vi "AwakeRunner.vi"() -> ()   [LabVIEW 2012]
uses:
  <vilib>/vision/Image Controls.llb/IMAQ Image.ctl
  <vilib>/Platform/TimedLoop/XDataNode/timing_clust.ctl
  <vilib>/Platform/TimedLoop/XDataNode/nitl_modes.ctl
  <vilib>/Platform/TimedLoop/XDataNode/wakeup.ctl
  <instrlib>/niHWS/nihws.llb/niHWS Open File Permissions ID.ctl
  <vilib>/Instr/_visa.llb/Select Event Type.ctl
  <vilib>/DAQmx/write.llb/DAQmx Write (Digital Bool 1Line 1Point).vi
  <vilib>/DAQmx/read.llb/DAQmx Read (Analog Wfm 1Chan NSamp).vi
  <instrlib>/niHWS/nihws.llb/niHWS Write Analog DBL.vi
  <instrlib>/niHWS/nihws.llb/niHWS Write Analog WDT.vi
  <vilib>/DAQmx/miscellaneous.llb/DAQmx Fill In Error Info.vi
  <vilib>/platform/TimedLoop/XDataNode/XDataNode.xnode
  <vilib>/express/express arith-compare/Formula/XNode/ExpressFormulaBlockNode.xnode
  <resource>/objmgr/daqmx.rc
  <vilib>/vision/NI_Vision_Development_Module.lvlib
  <vilib>/ptbypt/NI_PtbyPt.lvlib
  <vilib>/Platform/TimedLoop/XDataNode/XDNodeRunTimeDep.lvlib
panel:
  out "Numeric 2":i32
  out "Numeric":i32
  in  "SyncWrite":bool
  out "Click Value":i8
  out "Image Dst Out":T1
  out "Ephys Rate":dbl=1000.0
  out "Waveform Chart":waveform(dbl)(graph)
  out "Speed History":dbl(graph)
  in  "Magnify":bool
  in  "stop":bool
  out "Camera":T1(plugin-control)
  out "Rec Time":dbl format="%#_3g"
  out "fps":dbl format="%#_2g"
  in  "Rec":bool
  in  "Path":path
  in  "Gain":dbl(slide)=2.6607250597988097 min=1.0 max=3.9810717055349722 scale=0.0..4.0
  in  "Exposure Time":dbl(slide)=16602.0 min=56.0 max=16602.0 scale=0.0..16600.0
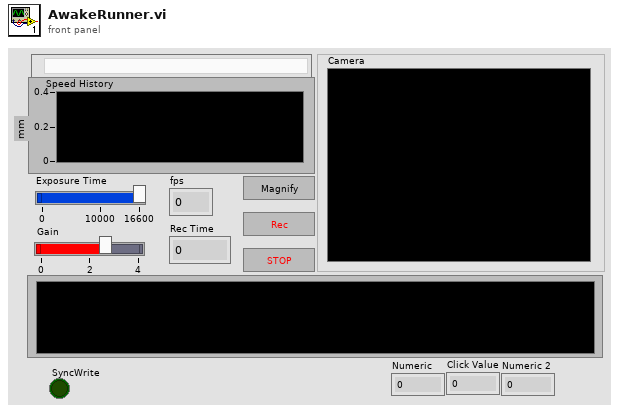
[diagram p1: front panel]
types:
  T1 = typedef "IMAQ Image.ctl" = refnum<image>
  T2 = typedef "XDNodeRunTimeDep.lvlib/timing_clust.ctl" = cluster{"Expected End [f-1]":u64, "Actual End [f-1]":u64, "Finished Late? [f-1]":bool, "Expected End [i-1]":u64, "Actual End [i-1]":u64, "Finished Late? [i-1]":bool, "Expected Start [i]":u64, "Actual Start [i]":u64, "Expected Start [f]":u64, "Actual Start [f]":u64, "Source Name":string, "Structure Name":string, "Period":i64, "Deadline":i64, "Offset":i64, "Start":i64, "Priority":i32, "Timeout":i32, "Mode":T3, "Wakeup Reason":T4, "Error":errorcluster, "Source Type":string, "Secondary Source Type":string, "Global End Time":u64, "Global Start Time":u64, "Frame Duration":u64, "Iteration Duration":u64, "Assigned CPU":i32, "I/O Scan Engine Mode":u32}
  T3 = typedef "XDNodeRunTimeDep.lvlib/nitl_modes.ctl" = enum32{"No Change", "Process missed periods, maintain original phase", "Discard missed periods, maintain original phase", "Process missed periods, ignore original phase", "Discard missed periods, ignore original phase"}
  T4 = typedef "XDNodeRunTimeDep.lvlib/wakeup.ctl" = enum32{"Normal", "Aborted", "Asynchronous wakeup", "Timing source error", "Timed loop error", "Timeout"}
  T5 = enum32{"Invalid", "Standard", "Closed", "Hidden", "Minimized", "Maximized"}
  T6 = typedef "niHWS Open File Permissions ID.ctl" = enum32{"Read Only", "Read/Write Existing", "Read/Write/Create New", "Read/Write/Create New Always"}
  T7 = typedef "AviRefnum.ctl" = refnum<k1>
  T8 = typedef "Select Event Type.ctl" = u32
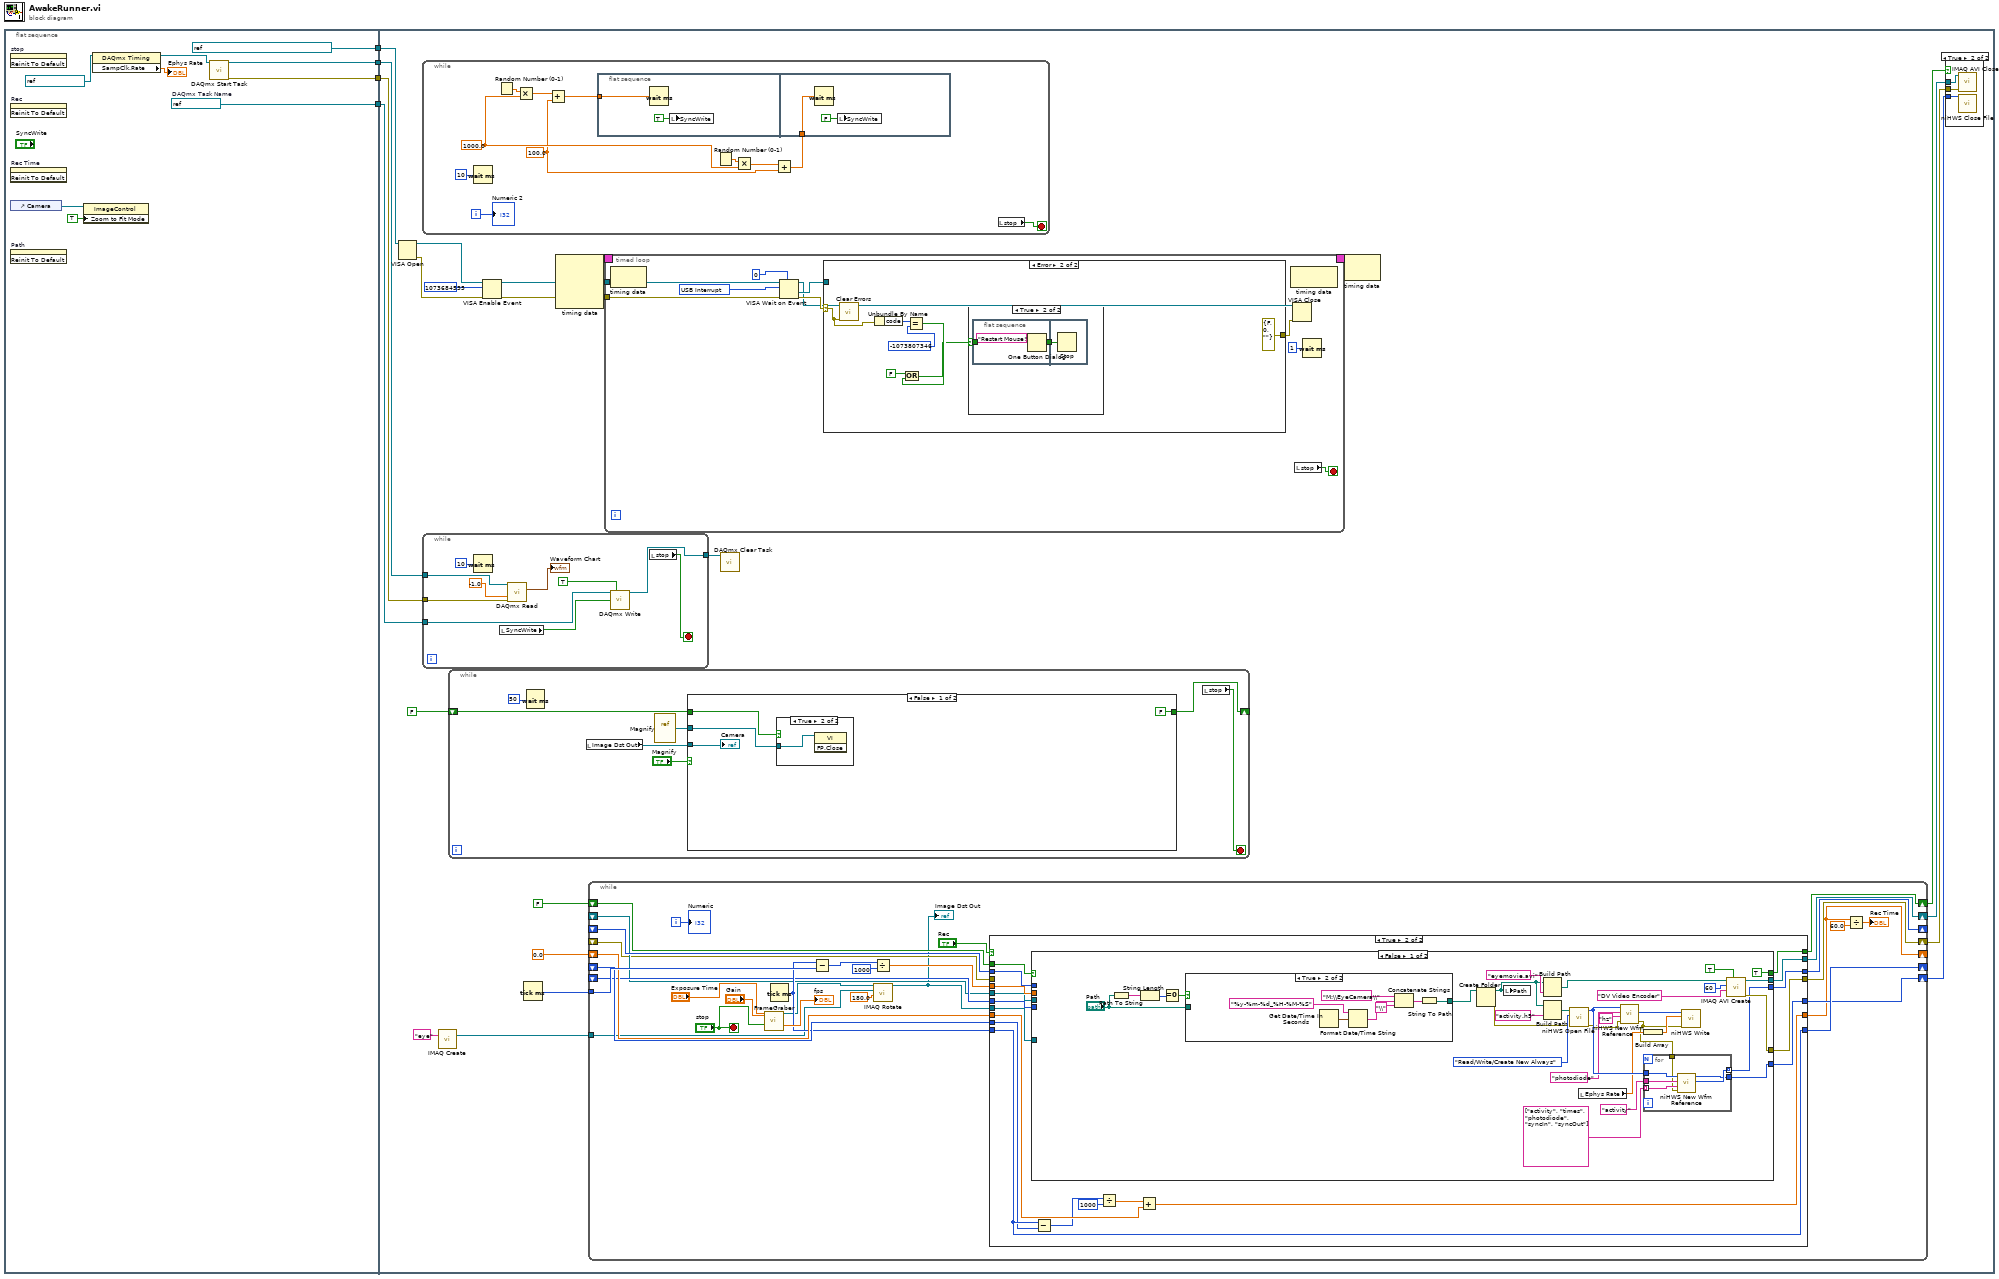
[diagram p0: block diagram]
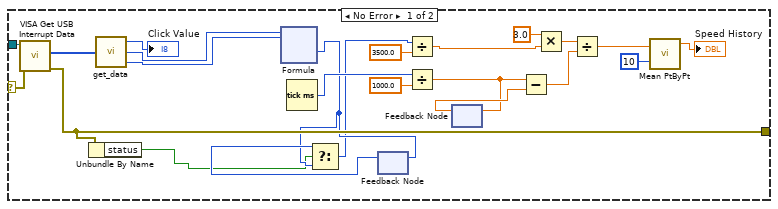
[diagram p2: hidden frame]
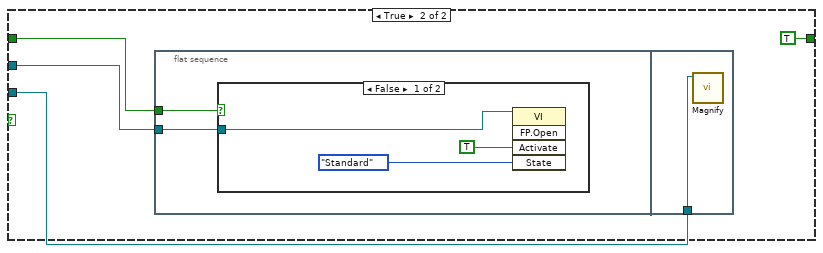
[diagram p5: hidden frame]
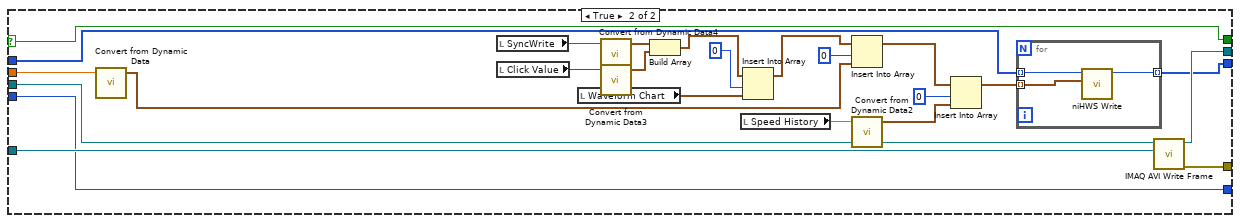
[diagram p10: hidden frame]
diagram:
  n1 = flat-sequence {
    tunnel: [w11] -> w4
    tunnel: [w10] -> w3
    tunnel: [refnum<visa-resource-name> "USB0::0x1532::0x0016::NI-VISA-1::RAW" ("VISA resource name")] -> w2
    tunnel: [w6] -> w1
    tunnel: w4 -> [w27]
    tunnel: w3 -> [w26]
    tunnel: w2 -> [w18]
    tunnel: w1 -> [w17]
    frame #0 {
      w6 = refnum<k21> "DigitalSync"  # DAQmx Task Name
      n2 = invoke on="stop" class="Bool (strict)" method="Reinit To Default"() -> ()  [unwired: 3 in, 3 out]
      n3 = invoke on="Rec" class="Bool (strict)" method="Reinit To Default"() -> ()  [unwired: 3 in, 3 out]
      n4 = invoke on="Rec Time" class="DigNum (strict)" method="Reinit To Default"() -> ()  [unwired: 3 in, 3 out]
      n5 = control-ref of="Camera"() -> (w13:refnum<vi>)
      n6 = invoke on="Path" class="Path" method="Reinit To Default"() -> ()  [unwired: 3 in, 3 out]
      n7 = property on="Property Node" class="ImageControl"(reference=w13, "Zoom to Fit Mode"=TRUE) -> ()  [unwired: 1 in, 2 out]
      n8 = property class="DAQmx Timing"(reference=refnum<k21> "PhotodiodeBall" ("task/channels in")) -> (reference out=w7:refnum<k21>, "SampClk.Rate"=→"Ephys Rate":dbl)  [unwired: 1 in, 1 out]
      n9 = call <vilib>:"DAQmx Start Task.vi"("task/channels in"=w7) -> ("task out"=w11:refnum<k21>, "error out"=w10:errorcluster)  [unwired: 13 in]
    }
    frame #1 {
      n10 = VISA Open(VISA resource name=w18) -> (VISA resource name=w23:refnum<visa-resource-name>, error out=w22:errorcluster)  [unwired: 1 in, 3 out]
      n11 = while {
        i -> [w95]
        stop <- w97 stop-if-true
        w98 = 100.0 ("y")
        w99 = 1000.0 ("y")
        n12 = Wait (ms)(milliseconds to wait=u32 10) -> ()  [unwired: 1 out]
        n13 = Random Number (0-1)() -> (number: 0 to 1=w105:dbl)
        n14 = Multiply(x=w105, y=w99) -> (x*y=w104:dbl)
        n15 = Add(x=w104, y=w98) -> (x+y=w103:dbl)
        n16 = flat-sequence {
          tunnel: w103 -> [w106]
          tunnel: w100 -> [w108]
          frame #0 {
            n17 = Wait (ms)(milliseconds to wait=w106) -> ()  [unwired: 1 out]
            n18 = local write "SyncWrite"(TRUE ("data")) -> ()
          }
          frame #1 {
            n19 = Wait (ms)(milliseconds to wait=w108) -> ()  [unwired: 1 out]
            n20 = local write "SyncWrite"(FALSE ("data")) -> ()
          }
        }
        n21 = Random Number (0-1)() -> (number: 0 to 1=w101:dbl)
        n22 = Multiply(x=w101, y=w99) -> (x*y=w102:dbl)
        n23 = Add(x=w102, y=w98) -> (x+y=w100:dbl)
        n24 = local read "stop"() -> (w97:bool)
        "Numeric 2" <- w95
      }
      n25 = while {
        tunnel: w27 -> [w118]
        tunnel: w26 -> [w117]
        tunnel: w17 -> [w112]
        tunnel: [w111] -> w16
        stop <- w119 stop-if-true
        n26 = Wait (ms)(milliseconds to wait=u32 10) -> ()  [unwired: 1 out]
        n27 = local read "SyncWrite"() -> (w110:bool)
        n28 = call-poly <vilib>:"DAQmx Read.vi"("task/channels in"=w118, "timeout"=-1.0, "error in"=w117) -> ("data"=→"Waveform Chart":waveform(dbl))  [unwired: 10 in, 2 out]
        n29 = call-poly <vilib>:"DAQmx Write.vi"("task/channels in"=w112, "auto start"=TRUE, "data"=w110) -> ("task out"=w111:refnum<k21>)  [unwired: 10 in, 2 out]
        n30 = local read "stop"() -> (w119:bool)
      }
      n31 = call "IMAQ Create"("Image Name"="eye") -> ("New Image"=w19:T1)  [unwired: 4 in, 1 out]
      n32 = while {
        shift-right: [w123] -> _
        shift-left: FALSE -> [w122]
        stop <- w124 stop-if-true
        n33 = Wait (ms)(milliseconds to wait=u32 50) -> ()  [unwired: 1 out]
        n34 = local read "Image Dst Out"() -> (w120:T1)
        n35 = vi-ref "Magnify.vi"() -> (w126:refnum<vi>)
        n36 = case shown="False" "Magnify" {
          tunnel: w126 -> [w130 w135]
          tunnel: [FALSE TRUE] -> w123
          tunnel: w122 -> [w129 w133]
          tunnel: w120 -> [w127 w132]
          frame False {
            n37 = case shown="True" w129 {
              tunnel: w130 -> [_ w131]
              frame False {
              }
              frame True {
                n38 = invoke class="VI" method="FP.Close"(reference=w131) -> ()  [unwired: 2 in, 3 out]
              }
            }
            "Camera" <- w127
          }
          frame True {
            n39 = flat-sequence {
              tunnel: w135 -> [w137]
              tunnel: w133 -> [w136]
              tunnel: w132 -> [w141]
              frame #0 {
                n40 = case shown="False" w136 {
                  tunnel: w137 -> [w139 _]
                  frame False {
                    n41 = invoke class="VI" method="FP.Open"(reference=w139, "Activate"=TRUE ("Wait Until Done"), "State"=T5."Standard") -> ()  [unwired: 2 in, 5 out]
                  }
                  frame True {
                  }
                }
              }
              frame #1 {
                n42 = call "Magnify.vi"("Camera 2"=w141) -> ()  [unwired: 11 in]
              }
            }
          }
        }
        n43 = local read "stop"() -> (w124:bool)
      }
      n44 = VISA Enable Event(8:w22, 10:u32 1073684535 ("event type"), 11:w23) -> (0:w25:errorcluster, 3:w24:refnum<visa-resource-name>)  [unwired: 1 out]
      n45 = Tick Count (ms)() -> (millisecond timer value=w32:u32)
      n46 = node-c288() -> (w15:T2)  [unwired: 4 in]
      n47 = while {
        tunnel: w32 -> [w174]
        shift-right: [w173] -> _
        shift-left: _ -> [w172]
        shift-right: [w153] -> _
        shift-left: 0.0 -> [w171]
        shift-right: [w161] -> w30
        shift-left: FALSE -> [w162]
        shift-right: [w158] -> _
        shift-left: _ -> [w157]
        shift-right: [w159] -> w29
        shift-left: _ -> [w156]
        shift-right: [w175] -> w35
        shift-left: _ -> [w155]
        shift-right: [w146] -> w34
        shift-left: _ -> [w154]
        tunnel: w19 -> [w147]
        i -> [w145]
        stop <- "stop" stop-if-true
        n48 = call "FrameGraber.vi"("Exposure Time"="Exposure Time", "Gain"="Gain", "Stop (F)"="stop") -> ("Image Out"=w150:T1, "Frame Rate"=→"fps":dbl)  [unwired: 20 in, 3 out]
        n49 = Tick Count (ms)() -> (millisecond timer value=w163:u32)
        n50 = Subtract(x=w163, y=w174) -> (x-y=w166:u32)
        n51 = Divide(x=w166, y=1000) -> (x/y=w164:dbl)
        n52 = call "IMAQ Rotate"("Angle (degrees)"=sgl 180.0, "Image Dst"=w147, "Image Src"=w150) -> ("Image Dst Out"=w149:T1)  [unwired: 7 in, 1 out]
        "Image Dst Out" <- w149
        n53 = case shown="True" "Rec" {
          tunnel: [w177 w191] -> w175
          tunnel: [w176 w190] -> w146
          tunnel: [w181 w197] -> w153
          tunnel: w164 -> [_ w188]
          tunnel: [w182 w200] -> w173
          tunnel: w163 -> [w182 w200]
          tunnel: w172 -> [_ w199]
          tunnel: w171 -> [w181 w198]
          tunnel: w149 -> [_ w189]
          tunnel: w162 -> [w180 w193]
          tunnel: [w180 w192] -> w161
          tunnel: [w178 w187] -> w159
          tunnel: [w179 w186] -> w158
          tunnel: w157 -> [w179 w185]
          tunnel: w156 -> [w178 w184]
          tunnel: w155 -> [w177 w183]
          tunnel: w154 -> [w176 _]
          frame False {
          }
          frame True {
            n54 = case shown="False" w193 {
              selector: w193 -> [_ w268]
              tunnel: [TRUE w268] -> w192
              tunnel: [w227 w267] -> w191
              tunnel: [w226 w266] -> w190
              tunnel: w189 -> [_ w265]
              tunnel: w188 -> [_ w261]
              tunnel: [w211 w264] -> w187
              tunnel: [w210 w253] -> w186
              tunnel: w185 -> [_ w254]
              tunnel: w184 -> [_ w264]
              tunnel: w183 -> [_ w263]
              frame False {
                n55 = Path To String(path="Path") -> (string=w228:string)
                n56 = String Length(string=w228) -> (length=w229:i32)
                n57 = Equal To 0?(x=w229) -> (x = 0?=w217:bool)
                n58 = case shown="True" w217 {
                  tunnel: [w237 w238] -> w215
                  tunnel: "Path" -> [w237 _]
                  frame False {
                  }
                  frame True {
                    n59 = Get Date/Time In Seconds() -> (seconds since 1Jan1904=w244:timestamp)
                    n60 = Format Date/Time String(time format string (%c)="%y-%m-%d_%H-%M-%S", seconds (now)=w244) -> (date/time string=w241:string)  [unwired: 1 in]
                    n61 = Concatenate Strings("M:\\EyeCamera\\", w241, "\\" ("string")) -> (w239:string)
                    n62 = String To Path(string=w239) -> (path=w238:path)
                  }
                }
                n63 = Create Folder(path (use dialog)=w215) -> (created path=w214:path, error out=w203:errorcluster)  [unwired: 2 in, 1 out]
                n64 = local write "Path"(w214) -> ()
                n65 = Build Path(base path=w214, name or relative path="eyemovie.avi" ("search string")) -> (appended path=w220:path)
                n66 = Build Path(base path=w214, name or relative path="activity.h5" ("search string")) -> (appended path=w218:path)
                n67 = call <instrlib>:"niHWS Open File.vi"("error in (no error)"=w203, "permissions (0:read only)"=niHWS_Open_File_Permissions_ID."Read/Write/Create New Always", "file path"=w218) -> ("error out"=w202:errorcluster, "file handle"=w209:u32)  [unwired: 7 in]
                n68 = local read "Ephys Rate"() -> (w205:dbl)
                n69 = call <instrlib>:"niHWS New Wfm Reference.vi"("error in (no error)"=w202, "waveform name (empty)"="hz", "group name (empty)"="photodiode", "file handle in"=w209) -> ("error out"=w201:errorcluster, "waveform reference"=w206:u32)  [unwired: 5 in, 1 out]
                n70 = Build Array(w205) -> (w204:dbl[])
                n71 = for {
                  tunnel: w209 -> [w236]
                  tunnel: [w235] -> w210 mode=indexing
                  tunnel: "activity" ("group name (empty)") -> [w234]
                  tunnel: string[] ["activity", "times", "photodiode", "syncIn", "syncOut"] -> [w233] mode=indexing
                  tunnel: [w232] -> w211
                  tunnel: w201 -> [w231]
                  n72 = call <instrlib>:"niHWS New Wfm Reference.vi"("error in (no error)"=w231, "waveform name (empty)"=w233, "group name (empty)"=w234, "file handle in"=w236) -> ("waveform reference"=w235:u32, "file handle out"=w232:u32)  [unwired: 5 in, 1 out]
                }
                n73 = call-poly <instrlib>:"niHWS Write.vi"("error in (no error)"=w201, "data"=w204, "waveform reference in"=w206) -> ()  [unwired: 7 in, 2 out]
                n74 = call "IMAQ AVI Create"("Has Data"=TRUE, "Compression Filter"="DV Video Encoder" ("Compressor"), "Frames Per Second"=u32 60, "AVI Path"=w220) -> ("error out"=w226:errorcluster, "Avi Refnum"=w227:T7)  [unwired: 3 in, 3 out]
              }
              frame True {
                n75 = call "Convert from Dynamic Data"("Dynamic Data Type"=w261) -> ("Waveform"=w260:waveform(dbl))  [unwired: 3 in]
                n76 = local read "SyncWrite"() -> (w245:bool)
                n77 = local read "Click Value"() -> (w248:i8)
                n78 = local read "Waveform Chart"() -> (w250:waveform(dbl))
                n79 = call "Convert from Dynamic Data4"("Dynamic Data Type"=w245) -> ("Waveform"=w246:waveform(dbl))  [unwired: 3 in]
                n80 = call "Convert from Dynamic Data3"("Dynamic Data Type"=w248) -> ("Waveform"=w247:waveform(dbl))  [unwired: 3 in]
                n81 = Build Array(w246, w247) -> (w252:waveform(dbl)[])
                n82 = local read "Speed History"() -> (w257:dbl)
                n83 = Insert Into Array(array=w252, index=0, new element=w250) -> (w249:waveform(dbl)[])
                n84 = Insert Into Array(array=w249, index=0, new element=w260) -> (w258:waveform(dbl)[])
                n85 = call "Convert from Dynamic Data2"("Dynamic Data Type"=w257) -> ("Waveform"=w256:waveform(dbl))  [unwired: 3 in]
                n86 = Insert Into Array(array=w258, index=0, new element=w256) -> (w255:waveform(dbl)[])
                n87 = for {
                  tunnel: w254 -> [w271] mode=indexing
                  tunnel: w255 -> [w270] mode=indexing
                  tunnel: [w269] -> w253 mode=indexing
                  n88 = call-poly <instrlib>:"niHWS Write.vi"("analog waveform"=w270, "waveform reference in"=w271) -> ("waveform reference out"=w269:u32)  [unwired: 8 in, 1 out]
                }
                n89 = call "IMAQ AVI Write Frame"("Image"=w265, "Avi Refnum"=w263) -> ("error out"=w266:errorcluster, "Avi Refnum (duplicate)"=w267:T7)  [unwired: 8 in]
              }
            }
            n90 = Subtract(x=w200, y=w199) -> (x-y=w196:u32)
            n91 = Divide(x=w196, y=1000) -> (x/y=w194:dbl)
            n92 = Add(x=w194, y=w198) -> (x+y=w197:dbl)
          }
        }
        n93 = Divide(x=w153, y=60.0) -> (x/y=→"Rec Time":dbl)
        "Numeric" <- w145
      }
      n94 = timed-loop {
        tunnel: w24 -> [w45]
        tunnel: w25 -> [w36]
        timing: w15 -> [_]
        timing-out: [_] -> w14
        stop <- w42 stop-if-true
        w41 = T8 1073684535 items=["Service Request"=1073684491, "Trigger"=3221168138, "Clear"=1073684493, "VXI Signal"=1073684512, "VXI/VME Interrupt"=3221168161, "VXI/VME Sysfail"=1073684509, "VXI/VME Sysreset"=1073684510, "GPIB CIC"=1073684498, "GPIB Talk"=1073684499, "GPIB Listen"=1073684500, "PXI Interrupt"=1073684514, "Serial Break"=1073684515, "Serial TermChar"=1073684516, "Serial CTS"=1073684521, "Serial DSR"=1073684522, "Serial DCD"=1073684524, "Serial RI"=1073684526, "Serial Character"=1073684533, "USB Interrupt"=1073684535, "All Enabled"=1073709055] ("Event Type")
        n95 = node-c288() -> ()  [unwired: 1 in, 1 out]
        n96 = VISA Wait on Event(7:u32 0 ("timeout (0)"), 8:w36, 10:w41, 11:w45) -> (0:w39:errorcluster, 1:w44:refnum<visa-resource-name>, 3:w37:refnum<visa-resource-name>)  [unwired: 2 out]
        n97 = case shown="Error" w39 {
          selector: w39 -> [w53 w86]
          tunnel: [w52 errorcluster {"status"=FALSE, "code"=0, "source"=""} ("error out")] -> w38
          tunnel: w44 -> [w70 _]
          frame No Error {
            n98 = call <vilib>:"VISA Get USB Interrupt Data.vi"("error in (no error)"=w53, "VISA USB Intr Event"=w70) -> ("error out"=w52:errorcluster, "data buffer"=w69:u8[])  [unwired: 8 out]
            n99 = Unbundle By Name(w52) -> ("status"=w48:bool)
            n100 = call "get_data.vi"("data buffer"=w69) -> ("Click Value"=→"Click Value":i8, "X Value"=w54:i8, "Y Value"=w55:i8)
            n101 = xnode ("Formula")("X1"=w54, "X2"=w55) -> ("Result"=w50:i8)  [unwired: 1 in, 1 out]
            n102 = Tick Count (ms)() -> (millisecond timer value=w65:u32)
            n103 = feedback-in #1(w50) -> ()
            n104 = feedback #1() -> (w51:i8)  [unwired: 1 in]
            n105 = Select(t=w51, s=w48, f=w50) -> (s? t:f=w49:i8)
            n106 = Divide(x=w49, y=3500.0 ("DPI")) -> (x/y=w62:dbl)
            n107 = Divide(x=w65, y=1000.0) -> (x/y=w63:dbl)
            n108 = feedback #2() -> (w67:dbl)  [unwired: 1 in]
            n109 = feedback-in #2(w63) -> ()
            n110 = Subtract(x=w63, y=w67) -> (x-y=w66:dbl)
            n111 = Multiply(x=3.0, y=w62) -> (x*y=w61:dbl)
            n112 = Divide(x=w61, y=w66) -> (x/y=w58:dbl)
            n113 = call <vilib>:"Mean PtByPt.vi"("x"=w58, "sample length"=10) -> ("mean"=→"Speed History":dbl)  [unwired: 2 in, 1 out]
          }
          frame Error {
            n114 = call <vilib>:"Clear Errors.vi"("error in (no error)"=w86) -> ()  [unwired: 6 in, 1 out]
            n115 = Unbundle By Name(w86) -> ("code"=w82:i32)
            n116 = Equal?(x=w82, y=-1073807346) -> (x = y?=w84:bool)
            n117 = Or(x=FALSE, y=w84) -> (x .or. y?=w83:bool)
            n118 = case shown="True" w83 {
              selector: w83 -> [_ w89]
              frame False {
              }
              frame True {
                n119 = flat-sequence {
                  tunnel: w89 -> [w91]
                  tunnel: [w91] -> w88
                  tunnel: w88 -> [w92]
                  frame #0 {
                    n120 = One Button Dialog(message="Restart Mouse!") -> ()  [unwired: 1 in, 1 out]
                  }
                  frame #1 {
                    n121 = Stop(stop? (T)=w92) -> ()
                  }
                }
              }
            }
          }
        }
        n122 = node-c288() -> ()  [unwired: 1 in, 1 out]
        n123 = VISA Close(VISA resource name=w37, error in (no error)=w38) -> ()  [unwired: 1 out]
        n124 = local read "stop"() -> (w42:bool)
        n125 = Wait (ms)(milliseconds to wait=u32 1) -> ()  [unwired: 1 out]
      }
      n126 = call <vilib>:"DAQmx Clear Task.vi"("task in"=w16) -> ()  [unwired: 14 in, 1 out]
      n127 = node-c288(w14) -> ()  [unwired: 1 out]
      n128 = case shown="True" w30 {
        tunnel: w35 -> [_ w144]
        tunnel: w34 -> [_ w143]
        tunnel: w29 -> [_ w142]
        frame False {
        }
        frame True {
          n129 = call "IMAQ AVI Close"("error in (no error)"=w143, "Avi Refnum"=w144) -> ()  [unwired: 9 in, 1 out]
          n130 = call <instrlib>:"niHWS Close File.vi"("file handle"=w142) -> ()  [unwired: 10 in, 1 out]
        }
      }
    }
  }
